vi "Ex2-Calling the python-numpy.vi"() -> ()   [LabVIEW 2021]
uses:
  <vilib>/httpClient/LabVIEWHTTPClient.lvlib
panel:
  in  "Cluster":cluster{"Data":dbl[]}={"Data"=[1.8900125377989787, 1.5095488147320884, 1.483424194991855]} {"Data" format="%#.2g"}
  out "body":string="{\"Data\":[1.8900125377989787,1.5095488147320884,1.483424194991855]}"
  out "headers":string="HTTP/1.1 200 OK\r\ndate: Mon, 02 Mar 2026 11:10:48 GMT\r\nserver: uvicorn\r\ncontent-length: 66\r\ncontent-type: application/json\r\n\r\n"
  in  "url":string="http://localhost:8080/test_numpy"
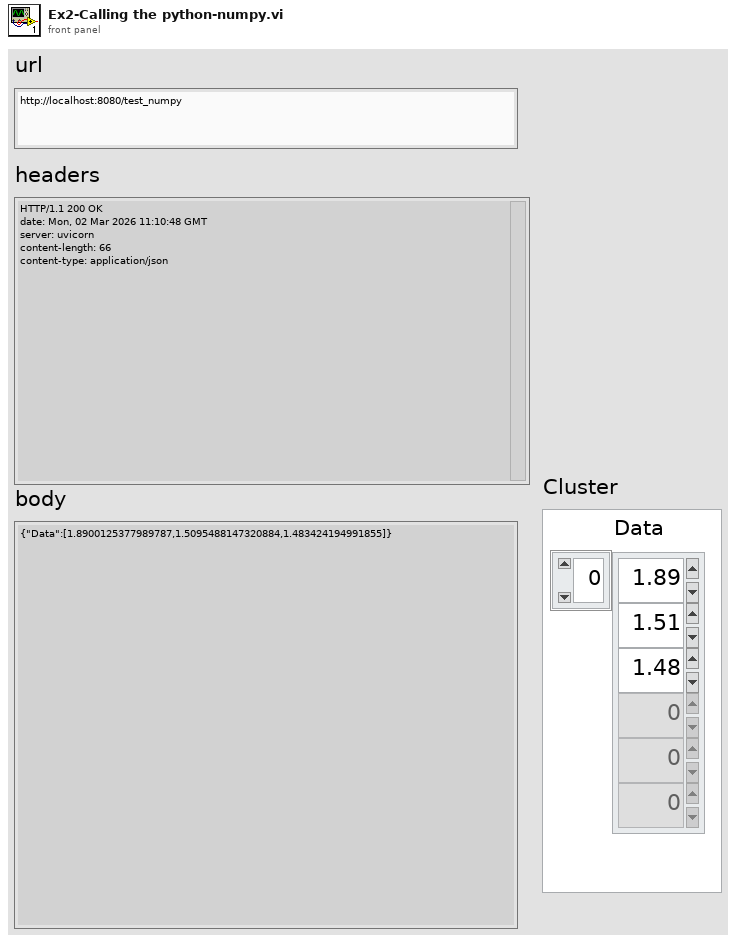
[diagram p1: front panel]
types:
  T1 = typedef "LabVIEWHTTPClient.lvlib/ClientHandle.ctl" = refnum<k1>
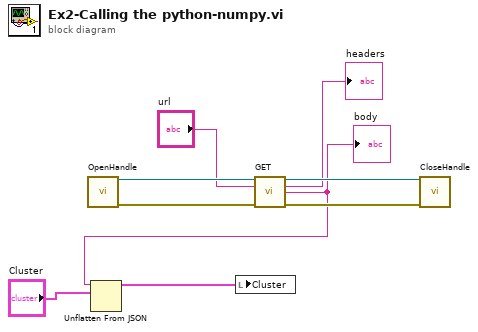
[diagram p0: block diagram]
diagram:
  n1 = call <vilib>:"OpenHandle.vi"() -> ("client handle out"=w9:T1, "error out"=w8:errorcluster)  [unwired: 14 in]
  n2 = call <vilib>:"GET.vi"("client handle"=w9, "url"="url", "error in (no error)"=w8) -> ("client handle out"=w7:T1, "headers"=→"headers":string, "body"=w3:string, "error out"=w6:errorcluster)  [unwired: 9 in]
  "body" <- w3
  n3 = Unflatten From JSON(JSON string=w3, type and defaults="Cluster") -> (value=w1:cluster{"Data":dbl[]})  [unwired: 5 in, 1 out]
  n4 = local write "Cluster"(w1) -> ()
  n5 = call <vilib>:"CloseHandle.vi"("client handle"=w7, "error in (no error)"=w6) -> ()  [unwired: 13 in, 1 out]
